vi "Global 1.vi"() -> ()   [LabVIEW 2015]
panel:
  out "BLE Packet (buf)":u8[](array[numeric])
  out "BLE Packet (data)":u8[][](array[numeric])
  out "BLE Packet":bool=TRUE
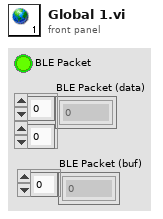
[diagram p1: front panel]
diagram:
